vi "全局键盘记录器.vi"() -> ()   [LabVIEW 2012]
uses:
  <vilib>/Utility/inputDevices.llb/closeKeyboard.vi
  <vilib>/Utility/inputDevices.llb/keyboardAcquire.vi
panel:
  out "记录中":bool
  in  "停止记录":bool
  in  "记录":bool
  out "记录键盘":T1(array[ring])
  in  "停止":bool
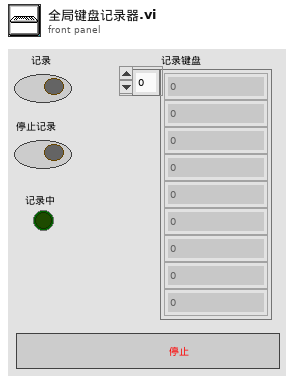
[diagram p1: front panel]
types:
  T1 = enum16{"0", "1", "2", "3", "4", "5", "6", "7", "8", "9", "A", "B", "C", "D", "E", "F", "G", "H", "I", "J", "K", "L", "M", "N", "O", "P", "Q", "R", "S", "T", "U", "V", "W", "X", "Y", "Z", "F1", "F2", "F3", "F4", "F5", "F6", "F7", "F8", "F9", "F10", "F11", "F12", "F13", "F14", "F15", "ADD", "BACK", "BACKSLASH", "CAPITAL", "COMMA", "DECIMAL", "DELETE", "DIVIDE", "DOWN", "END", "EQUALS", "ESCAPE", "GRAVE (`)", "HOME", "INSERT", "LBRACKET", "LCONTROL", "LEFT", "L ALT", "LSHIFT", "LWIN", "MINUS", "MULTIPLY", "NEXT", "NUMLOCK", "NUMPAD_0", "NUMPAD_1", "NUMPAD_2", "NUMPAD_3", "NUMPAD_4", "NUMPAD_5", "NUMPAD_6", "NUMPAD_7", "NUMPAD_8", "NUMPAD_9", "PAUSE", "PERIOD", "PRIOR (PG UP)", "RBRACKET", "RCONTROL", "RETURN", "RIGHT", "R ALT", "RSHIFT", "RWIN", "SCROLL", "SEMICOLON", "SLASH", "SPACE", "SUBTRACT", "TAB", "UP", "ENTER (num pad)", "' (quote)"}[]
  T2 = typedef "堆栈操作.ctl" = enum16{"初始化（Init）", "进栈（Push）", "出栈（Pop）", "状态（Status)", "释放"}
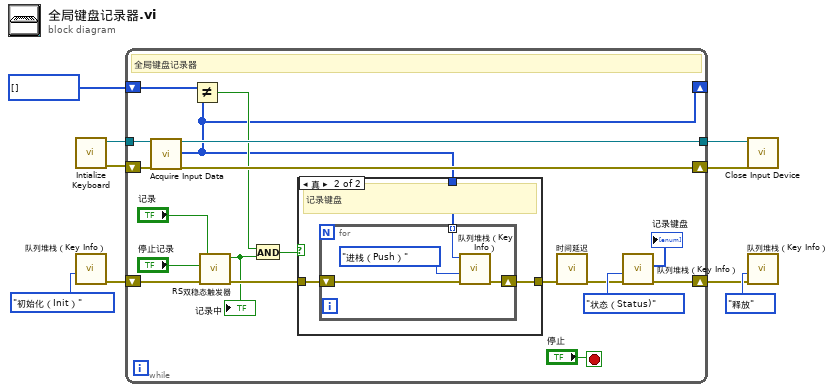
[diagram p0: block diagram]
diagram:
  w2 = T1 [] items=["0", "1", "2", "3", "4", "5", "6", "7", "8", "9", "A", "B", "C", "D", "E", "F", "G", "H", "I", "J", "K", "L", "M", "N", "O", "P", "Q", "R", "S", "T", "U", "V", "W", "X", "Y", "Z", "F1", "F2", "F3", "F4", "F5", "F6", "F7", "F8", "F9", "F10", "F11", "F12", "F13", "F14", "F15", "ADD", "BACK", "BACKSLASH", "CAPITAL", "COMMA", "DECIMAL", "DELETE", "DIVIDE", "DOWN", "END", "EQUALS", "ESCAPE", "GRAVE (`)", "HOME", "INSERT", "LBRACKET", "LCONTROL", "LEFT", "L ALT", "LSHIFT", "LWIN", "MINUS", "MULTIPLY", "NEXT", "NUMLOCK", "NUMPAD_0", "NUMPAD_1", "NUMPAD_2", "NUMPAD_3", "NUMPAD_4", "NUMPAD_5", "NUMPAD_6", "NUMPAD_7", "NUMPAD_8", "NUMPAD_9", "PAUSE", "PERIOD", "PRIOR (PG UP)", "RBRACKET", "RCONTROL", "RETURN", "RIGHT", "R ALT", "RSHIFT", "RWIN", "SCROLL", "SEMICOLON", "SLASH", "SPACE", "SUBTRACT", "TAB", "UP", "ENTER (num pad)", "' (quote)"] ("keys pressed")
  n1 = call <vilib>:"Intialize Keyboard.vi"() -> ("error out"=w9:errorcluster, "device ID"=w8:refnum<k1>)  [unwired: 10 in]
  n2 = call "队列堆栈（Key Info）.vi"("堆栈操作"=堆栈操作."初始化（Init）") -> ("error out"=w4:errorcluster)  [unwired: 7 in, 3 out]
  n3 = while {
    shift-right: [w19] -> w7
    shift-left: w9 -> [w27]
    tunnel: w8 -> [w28]
    tunnel: [w25] -> w6
    shift-right: [w10] -> w1
    shift-left: w4 -> [w22]
    shift-right: [w14] -> _
    shift-left: w2 -> [w18]
    stop <- "停止" stop-if-true
    # "全局键盘记录器"
    n4 = call-poly <vilib>:"Acquire Input Data.vi"("device ID"=w28, "error in (no error)"=w27) -> ("device ID"=w25:refnum<k1>, "keys pressed"=w14:T1, "error out"=w19:errorcluster)  [unwired: 15 in]
    n5 = Not Equal?(x=w18, y=w14) -> (x != y?=w16:bool)
    n6 = call "RS双稳态触发器.vi"("error in"=w22, "reset"="停止记录", "set"="记录") -> ("error out"=w21:errorcluster, "output"=w17:bool)  [unwired: 7 in]
    "记录中" <- w17
    n7 = And(x=w16, y=w17) -> (x .and. y?=w15:bool)
    n8 = case shown="真" w15 {
      tunnel: w14 -> [_ w30]
      tunnel: [w29 w32] -> w20
      tunnel: w21 -> [w29 w31]
      frame False {
      }
      frame True {
        # "记录键盘"
        n9 = for {
          shift-right: [w34] -> w32
          shift-left: w31 -> [w36]
          tunnel: w30 -> [w33] mode=indexing
          n10 = call "队列堆栈（Key Info）.vi"("error in (no error)"=w36, "堆栈操作"=堆栈操作."进栈（Push）", "入栈元素"=w33) -> ("error out"=w34:errorcluster)  [unwired: 5 in, 3 out]
        }
      }
    }
    n11 = call "时间延迟"("error in (no error)"=w20) -> ("error out"=w11:errorcluster)  [unwired: 10 in]
    n12 = call "队列堆栈（Key Info）.vi"("error in (no error)"=w11, "堆栈操作"=堆栈操作."状态（Status)") -> ("error out"=w10:errorcluster, "入栈所有元素"=→"记录键盘":T1)  [unwired: 6 in, 2 out]
  }
  n13 = call-poly <vilib>:"Close Input Device.vi"("error in (no error)"=w7, "device ID"=w6) -> ()  [unwired: 8 in, 1 out]
  n14 = call "队列堆栈（Key Info）.vi"("error in (no error)"=w1, "堆栈操作"=堆栈操作."释放") -> ()  [unwired: 6 in, 4 out]
